vi "libssh2_channel_set_blocking.vi"(8 "error in (no error)":errorcluster, 10 "blocking":bool, 11 "channel":T1) -> (0 "error out":errorcluster)   [LabVIEW 2013, in "libssh2.lvlib"]
doc: "Set blocking mode on a channel. This will affect the session and all channels.\n\nIf a read is performed on a channel with no data currently available, a blocking channel will wait for data to arrive and return what it received. A non-blocking channel will return immediately with an empty buffer. If a write is performed on a channel with no room for more data, a blocking channel will wait for room. A non-blocking channel will return immediately without writing anything."
uses:
  libssh2.lvlib
  Channel Refnum.ctl
  Not A Channel.vi
  <vilib>/Utility/error.llb/Error Cluster From Error Code.vi
  Global Settings.vi
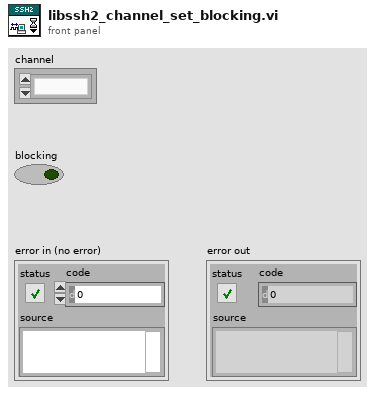
[diagram p1: front panel]
types:
  T1 = typedef "libssh2.lvlib/Channel Refnum.ctl" = refnum<k1>
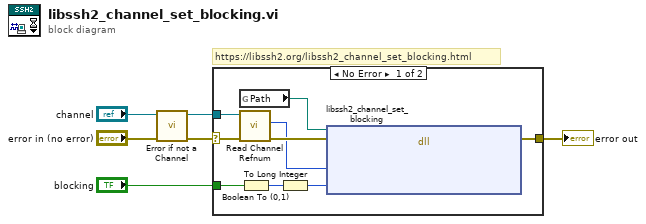
[diagram p0: block diagram]
diagram:
  # "https://libssh2.org/libssh2_channel_set_blocking.html"
  n1 = call "Error if not a Channel.vi"("error in (no error)"="error in (no error)", "channel"="channel") -> ("error out"=w3:errorcluster, "channel out"=w1:T1)  [unwired: 8 in]
  n2 = case shown="No Error" w3 {
    selector: w3 -> [w13 w16]
    tunnel: [w15 w16] -> w6
    tunnel: "blocking" -> [w14 _]
    tunnel: w1 -> [w12 _]
    frame No Error {
      n3 = global read "Global Settings.vi" "Path"() -> (w9:path)
      n4 = call "Read Channel Refnum.vi"("error in (no error)"=w13, "channel"=w12) -> ("error out"=w11:errorcluster, "LIBSSH2_CHANNEL*"=w10:u64)  [unwired: 8 in]
      n5 = Boolean To (0,1)(Boolean=w14) -> (0, 1=w8:i16)
      n6 = To Long Integer(number=w8) -> (32bit integer=w7:i32)
      n7 = dll-call lib="?" fn="libssh2_channel_set_blocking"(path in=w9, error in=w11, "channel"=w10, "blocking"=w7) -> (error out=w15:errorcluster)  [unwired: 4 in, 1 out]
    }
    frame Error {
    }
  }
  "error out" <- w6
